vi "set_params.vi"(0 "dummyStage in":refnum<class "dummyStage.lvclass">, 3 "error in (no error)":errorcluster) -> (7 "dummyStage out":refnum<class "dummyStage.lvclass">, 10 "error out":errorcluster)   [LabVIEW 2019, in "dummyStage.lvlib" / "dummyStage.lvclass"]
uses:
  dummyStage.lvclass
panel:
  in  "OK Button":bool
  in  "pos_max":dbl[](array[numeric])=[10000.0]
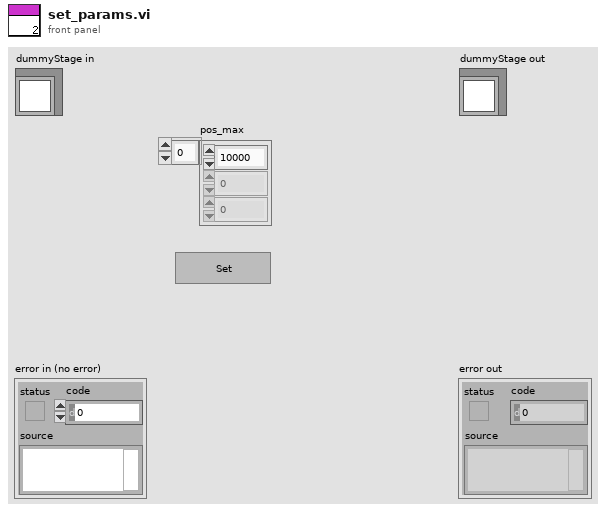
[diagram p1: front panel]
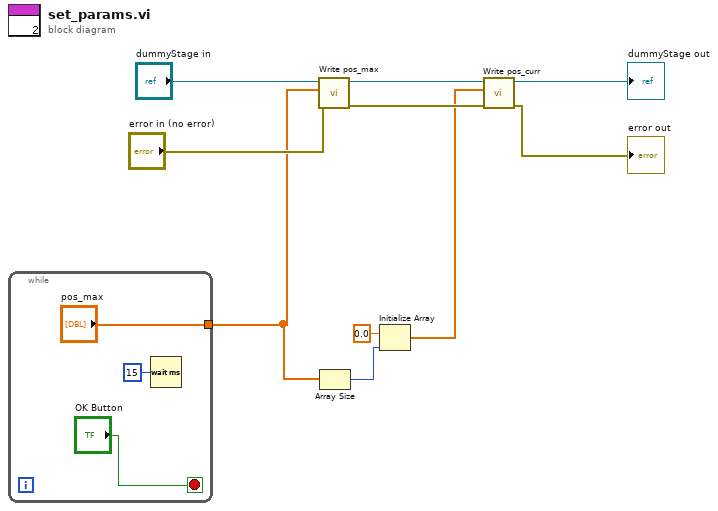
[diagram p0: block diagram]
diagram:
  n1 = while {
    tunnel: ["pos_max"] -> w3
    stop <- "OK Button" stop-if-true
    n2 = Wait (ms)(milliseconds to wait=u32 15) -> ()  [unwired: 1 out]
  }
  n3 = call-dynamic "Write pos_max.vi"("error in (no error)"="error in (no error)", "pos_max"=w3, "_stage in"="dummyStage in") -> ("error out"=w6:errorcluster, "_stage out"=w8:refnum<class "dummyStage.lvclass">)  [unwired: 7 in]
  n4 = Array Size(array=w3) -> (size(s)=w2:i32)
  n5 = Initialize Array(0.0 ("element"), w2) -> (w1:dbl[])
  n6 = call-dynamic "Write pos_curr.vi"("error in (no error)"=w6, "set_pos"=w1, "_stage in"=w8) -> ("error out"=→"error out":errorcluster, "_stage out"=→"dummyStage out":refnum<class "dummyStage.lvclass">)  [unwired: 7 in]
